vi "Vacuum Manual Control.vi"() -> ()   [LabVIEW 2017]
uses:
  Shared Components/Gantry Class/Gantry Class.lvclass
  Shared Components/WorkTable Class/WorkTable Class.lvclass
panel:
  out "error out":errorcluster
  in  "Module Chuck 5-slot 4 status":bool=TRUE
  in  "Module Chuck 5-slot 3 status":bool=TRUE
  in  "Module Chuck 5-slot 2 status":bool=TRUE
  in  "Module Chuck 5-slot 1 status":bool=TRUE
  in  "Module Chuck 4-slot 4 status":bool=TRUE
  in  "Module Chuck 4-slot 3 status":bool=TRUE
  in  "Module Chuck 4-slot 2 status":bool=TRUE
  in  "Module Chuck 4-slot 1 status":bool=TRUE
  in  "Module Chuck 3 status":bool=TRUE
  in  "Module Chuck 2 status":bool=TRUE
  in  "Module Chuck 1 status":bool=TRUE
  in  "Weight Chuck status":bool=TRUE
  in  "Stamp Chuck status":bool=TRUE
  in  "Glue Resevoir Chuck status":bool=TRUE
  in  "Outer Gantry Head status":bool=TRUE
  in  "Inner Gantry Head status":bool=TRUE
  in  "Reset all to ON":bool
  in  "Reset all to OFF":bool
  in  "stop program":bool
  in  "Virtual Mode":bool
  in  "Config Folder":path=path "C:/Users/husker/Desktop/gantry/Config"
  # "Note:\nMay not always read the correct initial vacuum states, due to incorrect reading of the worktable.\nIf in doubt, change all to off!"
  # "Current\nState"
  # "Vacuum\nChannel"
  # "Inner Gantry Head"
  # "Outer Gantry Head"
  # "Glue Resevoir Chuck"
  # "Stamp Chuck"
  # "Weight Chuck"
  # "Module Chuck 1"
  # "Module Chuck 2"
  # "Module Chuck 3"
  # "Module Chuck 4\n\nSlot 1\n\nSlot 2\n\nSlot 3\n\nSlot 4"
  # "Module Chuck 5\n\nSlot 1\n\nSlot 2\n\nSlot 3\n\nSlot 4"
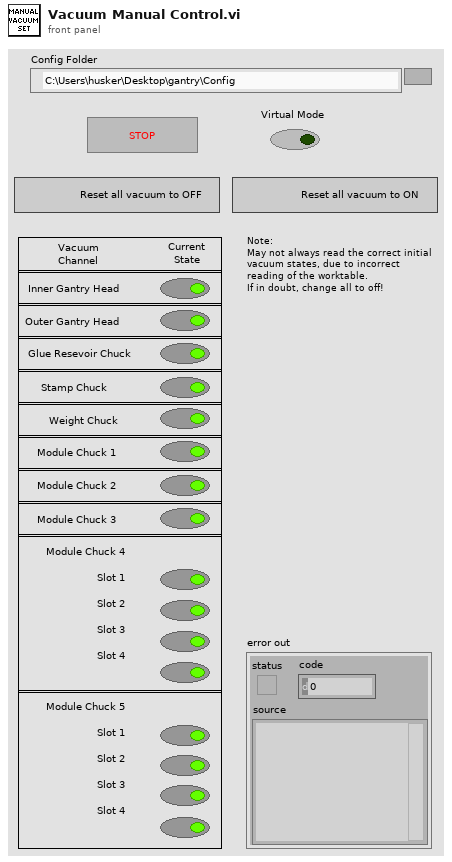
[diagram p1: front panel]
types:
  T1 = typedef "Worktable_Manifold.ctl" = cluster{"Vacuum Channel Status":T2[], "Vacuum Channel Names":T3[]}
  T2 = typedef "Worktable_Manifold Channel.ctl" = cluster{"Enabled":bool, "Hardware Path":string}
  T3 = typedef "Worktable_Manifold Channel Names.ctl" = cluster{"Channel Name":string, "Channel Number":i8}
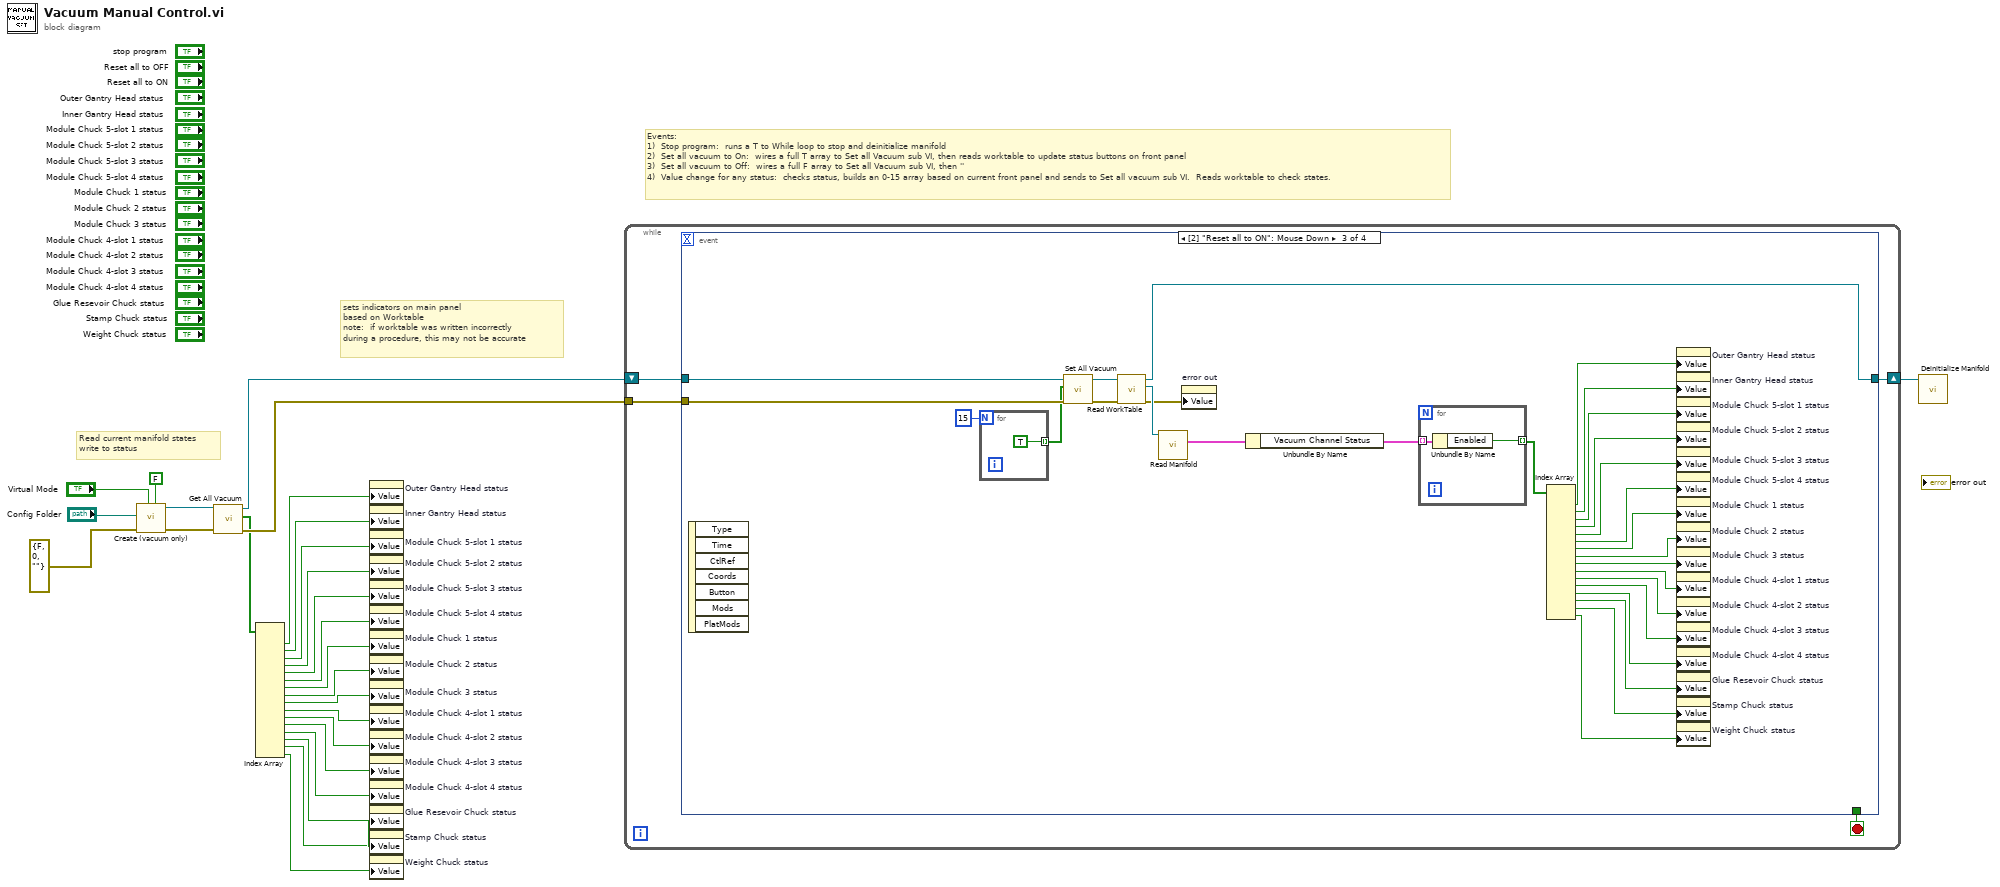
[diagram p0: block diagram]
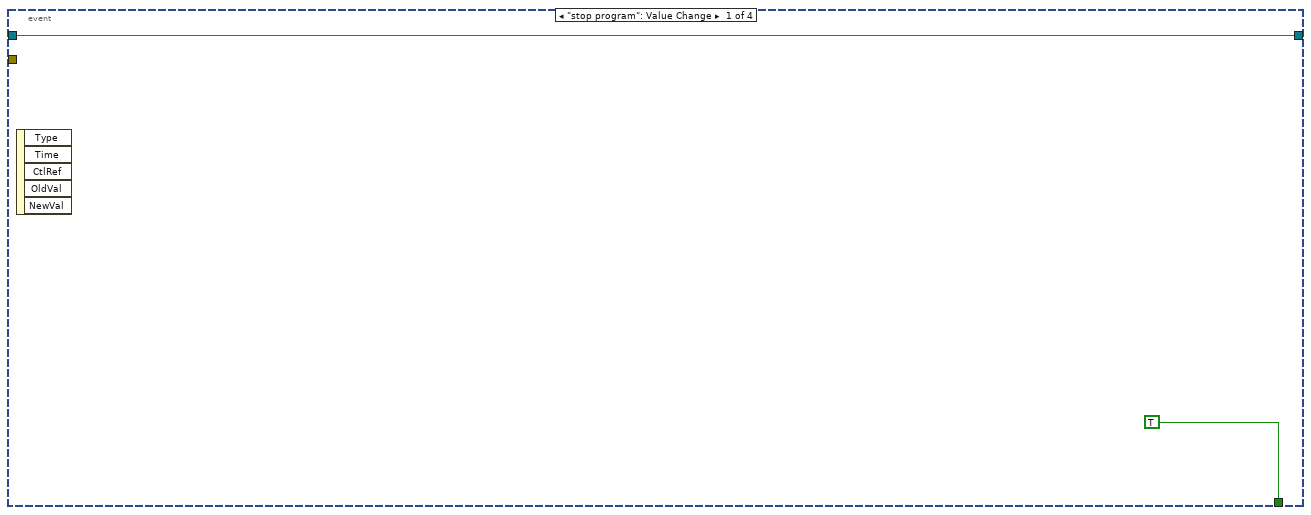
[diagram p2: hidden frame]
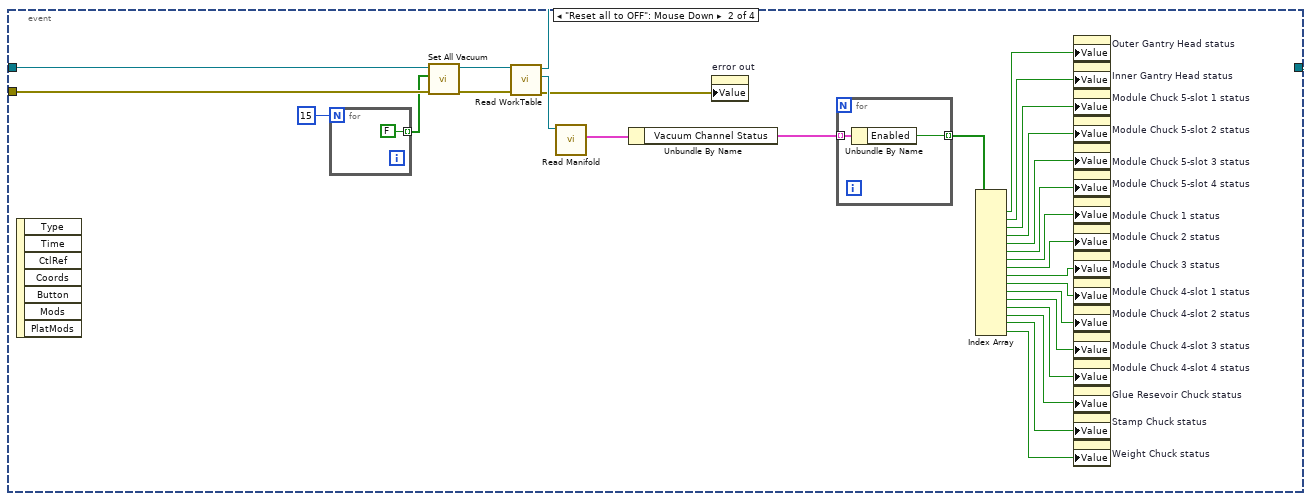
[diagram p3: hidden frame]
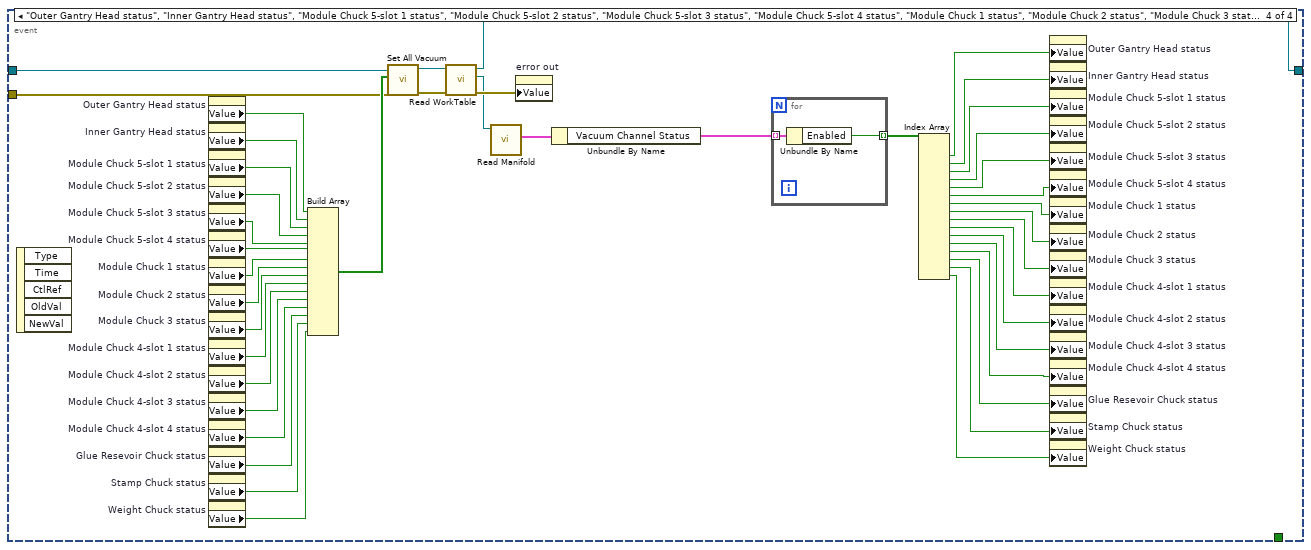
[diagram p4: hidden frame]
diagram:
  # "Events:\n1)  Stop program:  runs a T to While loop to stop and deinitialize manifold\n2)  Set all vacuum to On:  wires a full T array to Set all Vacuum sub VI, then reads worktable to update status buttons on front panel\n3)  Set all vacuum to Off:  wires a full F array to Set all Vacuum sub VI, then ''\n4)  Value change for any status:  checks status, builds an 0-15 array based on current front panel and sends to Set all vacuum sub VI.  Reads worktable to check states."
  # "sets indicators on main panel\nbased on Worktable\nnote:  if worktable was written incorrectly\nduring a procedure, this may not be accurate"
  # "Read current manifold states\nwrite to status"
  n1 = call "Create (vacuum only).vi"("Reset Vacuum to All Off?"=FALSE, "Virtual Mode"="Virtual Mode", "error in"=errorcluster {"status"=FALSE, "code"=0, "source"=""}, "Config Folder"="Config Folder") -> ("error out"=w14:errorcluster, "Gantry out"=w15:refnum<class "Gantry Class.lvclass">)  [unwired: 6 in]
  n2 = call "Get All Vacuum.vi"("error in"=w14, "Gantry Class in"=w15) -> ("error out"=w12:errorcluster, "Channel Array"=w11:bool[], "Gantry Class out"=w13:refnum<class "Gantry Class.lvclass">)  [unwired: 7 in]
  n3 = Index Array(array=w11) -> (element #1=w22:bool, element #2=w21:bool, element #3=w20:bool, element #4=w19:bool, element #5=w18:bool, element #6=w17:bool, element #7=w10:bool, element #8=w9:bool, element #9=w8:bool, element #10=w7:bool, element #11=w6:bool, element #12=w5:bool, element #13=w4:bool, element #14=w3:bool, element #15=w2:bool, element #16=w1:bool)  [unwired: 16 in]
  n4 = property on="Outer Gantry Head status" class="Bool (strict)"("Value"=w22) -> ()  [unwired: 2 in, 2 out]
  n5 = property on="Inner Gantry Head status" class="Bool (strict)"("Value"=w21) -> ()  [unwired: 2 in, 2 out]
  n6 = property on="Module Chuck 5-slot 1 status" class="Bool (strict)"("Value"=w20) -> ()  [unwired: 2 in, 2 out]
  n7 = property on="Module Chuck 5-slot 2 status" class="Bool (strict)"("Value"=w19) -> ()  [unwired: 2 in, 2 out]
  n8 = property on="Module Chuck 5-slot 3 status" class="Bool (strict)"("Value"=w18) -> ()  [unwired: 2 in, 2 out]
  n9 = property on="Module Chuck 5-slot 4 status" class="Bool (strict)"("Value"=w17) -> ()  [unwired: 2 in, 2 out]
  n10 = property on="Module Chuck 1 status" class="Bool (strict)"("Value"=w10) -> ()  [unwired: 2 in, 2 out]
  n11 = property on="Module Chuck 2 status" class="Bool (strict)"("Value"=w9) -> ()  [unwired: 2 in, 2 out]
  n12 = property on="Module Chuck 3 status" class="Bool (strict)"("Value"=w8) -> ()  [unwired: 2 in, 2 out]
  n13 = property on="Module Chuck 4-slot 1 status" class="Bool (strict)"("Value"=w7) -> ()  [unwired: 2 in, 2 out]
  n14 = property on="Module Chuck 4-slot 2 status" class="Bool (strict)"("Value"=w6) -> ()  [unwired: 2 in, 2 out]
  n15 = property on="Module Chuck 4-slot 3 status" class="Bool (strict)"("Value"=w5) -> ()  [unwired: 2 in, 2 out]
  n16 = property on="Module Chuck 4-slot 4 status" class="Bool (strict)"("Value"=w4) -> ()  [unwired: 2 in, 2 out]
  n17 = property on="Glue Resevoir Chuck status" class="Bool (strict)"("Value"=w3) -> ()  [unwired: 2 in, 2 out]
  n18 = property on="Stamp Chuck status" class="Bool (strict)"("Value"=w2) -> ()  [unwired: 2 in, 2 out]
  n19 = property on="Weight Chuck status" class="Bool (strict)"("Value"=w1) -> ()  [unwired: 2 in, 2 out]
  n20 = while {
    tunnel: w12 -> [w28]
    shift-right: [w27] -> w16
    shift-left: w13 -> [w29]
    stop <- w30 stop-if-true
    n21 = event shown="[2] \"Reset all to ON\": Mouse Down" {
      selector: _ -> [_ _ _ _]
      dyn-events: _ -> [_ _ _ _]
      timeout: _ -> [_ _ _ _]
      tunnel: [TRUE _ _ _] -> w30
      tunnel: w29 -> [w31 w49 w80 w126]
      tunnel: w28 -> [_ w48 w79 w106]
      tunnel: [w31 w50 w78 w124] -> w27
      event "stop program": Value Change {
        n22 = event-data() -> ()  [unwired: 1 in, 5 out]
      }
      event "Reset all to OFF": Mouse Down {
        n23 = event-data() -> ()  [unwired: 1 in, 7 out]
        n24 = for {
          N: 15 -> [_]
          tunnel: [FALSE ("On/Off")] -> w46 mode=indexing
        }
        n25 = call "Set All Vacuum.vi"("error in"=w48, "Channel Array"=w46, "Gantry Class in"=w49) -> ("error out"=w44:errorcluster, "Gantry Class out"=w45:refnum<class "Gantry Class.lvclass">)  [unwired: 7 in]
        n26 = call-dynamic "Read WorkTable.vi"("error in"=w44, "Gantry Class in"=w45) -> ("error out"=w51:errorcluster, "WorkTable Class.lvclass"=w58:refnum<class "WorkTable Class.lvclass">, "Gantry Class out"=w50:refnum<class "Gantry Class.lvclass">)  [unwired: 7 in]
        n27 = call-dynamic "Read Manifold.vi"("WorkTable Class in"=w58) -> ("Manifold"=w60:T1)  [unwired: 8 in, 2 out]
        n28 = Unbundle By Name(w60) -> ("Vacuum Channel Status"=w59:T2[])
        n29 = property on="error out" class="Clust (strict)"("Value"=w51) -> ()  [unwired: 2 in, 2 out]
        n30 = for {
          tunnel: w59 -> [w63] mode=indexing
          tunnel: [w62] -> w43 mode=indexing
          n31 = Unbundle By Name(w63) -> ("Enabled"=w62:bool)
        }
        n32 = Index Array(array=w43) -> (element #1=w57:bool, element #2=w56:bool, element #3=w55:bool, element #4=w54:bool, element #5=w53:bool, element #6=w52:bool, element #7=w42:bool, element #8=w41:bool, element #9=w40:bool, element #10=w39:bool, element #11=w38:bool, element #12=w37:bool, element #13=w36:bool, element #14=w35:bool, element #15=w34:bool, element #16=w33:bool)  [unwired: 16 in]
        n33 = property on="Outer Gantry Head status" class="Bool (strict)"("Value"=w57) -> ()  [unwired: 2 in, 2 out]
        n34 = property on="Inner Gantry Head status" class="Bool (strict)"("Value"=w56) -> ()  [unwired: 2 in, 2 out]
        n35 = property on="Module Chuck 5-slot 1 status" class="Bool (strict)"("Value"=w55) -> ()  [unwired: 2 in, 2 out]
        n36 = property on="Module Chuck 5-slot 2 status" class="Bool (strict)"("Value"=w54) -> ()  [unwired: 2 in, 2 out]
        n37 = property on="Module Chuck 5-slot 3 status" class="Bool (strict)"("Value"=w53) -> ()  [unwired: 2 in, 2 out]
        n38 = property on="Module Chuck 5-slot 4 status" class="Bool (strict)"("Value"=w52) -> ()  [unwired: 2 in, 2 out]
        n39 = property on="Module Chuck 1 status" class="Bool (strict)"("Value"=w42) -> ()  [unwired: 2 in, 2 out]
        n40 = property on="Module Chuck 2 status" class="Bool (strict)"("Value"=w41) -> ()  [unwired: 2 in, 2 out]
        n41 = property on="Module Chuck 3 status" class="Bool (strict)"("Value"=w40) -> ()  [unwired: 2 in, 2 out]
        n42 = property on="Module Chuck 4-slot 1 status" class="Bool (strict)"("Value"=w39) -> ()  [unwired: 2 in, 2 out]
        n43 = property on="Module Chuck 4-slot 2 status" class="Bool (strict)"("Value"=w38) -> ()  [unwired: 2 in, 2 out]
        n44 = property on="Module Chuck 4-slot 3 status" class="Bool (strict)"("Value"=w37) -> ()  [unwired: 2 in, 2 out]
        n45 = property on="Module Chuck 4-slot 4 status" class="Bool (strict)"("Value"=w36) -> ()  [unwired: 2 in, 2 out]
        n46 = property on="Glue Resevoir Chuck status" class="Bool (strict)"("Value"=w35) -> ()  [unwired: 2 in, 2 out]
        n47 = property on="Stamp Chuck status" class="Bool (strict)"("Value"=w34) -> ()  [unwired: 2 in, 2 out]
        n48 = property on="Weight Chuck status" class="Bool (strict)"("Value"=w33) -> ()  [unwired: 2 in, 2 out]
      }
      event "Reset all to ON": Mouse Down {
        n49 = event-data() -> ()  [unwired: 1 in, 7 out]
        n50 = for {
          N: 15 -> [_]
          tunnel: [TRUE ("On/Off")] -> w76 mode=indexing
        }
        n51 = call "Set All Vacuum.vi"("error in"=w79, "Channel Array"=w76, "Gantry Class in"=w80) -> ("error out"=w81:errorcluster, "Gantry Class out"=w82:refnum<class "Gantry Class.lvclass">)  [unwired: 7 in]
        n52 = call-dynamic "Read WorkTable.vi"("error in"=w81, "Gantry Class in"=w82) -> ("error out"=w75:errorcluster, "WorkTable Class.lvclass"=w89:refnum<class "WorkTable Class.lvclass">, "Gantry Class out"=w78:refnum<class "Gantry Class.lvclass">)  [unwired: 7 in]
        n53 = call-dynamic "Read Manifold.vi"("WorkTable Class in"=w89) -> ("Manifold"=w91:T1)  [unwired: 8 in, 2 out]
        n54 = property on="error out" class="Clust (strict)"("Value"=w75) -> ()  [unwired: 2 in, 2 out]
        n55 = Unbundle By Name(w91) -> ("Vacuum Channel Status"=w90:T2[])
        n56 = for {
          tunnel: w90 -> [w94] mode=indexing
          tunnel: [w93] -> w74 mode=indexing
          n57 = Unbundle By Name(w94) -> ("Enabled"=w93:bool)
        }
        n58 = Index Array(array=w74) -> (element #1=w88:bool, element #2=w87:bool, element #3=w86:bool, element #4=w85:bool, element #5=w84:bool, element #6=w83:bool, element #7=w73:bool, element #8=w72:bool, element #9=w71:bool, element #10=w70:bool, element #11=w69:bool, element #12=w68:bool, element #13=w67:bool, element #14=w66:bool, element #15=w65:bool, element #16=w64:bool)  [unwired: 16 in]
        n59 = property on="Outer Gantry Head status" class="Bool (strict)"("Value"=w88) -> ()  [unwired: 2 in, 2 out]
        n60 = property on="Inner Gantry Head status" class="Bool (strict)"("Value"=w87) -> ()  [unwired: 2 in, 2 out]
        n61 = property on="Module Chuck 5-slot 1 status" class="Bool (strict)"("Value"=w86) -> ()  [unwired: 2 in, 2 out]
        n62 = property on="Module Chuck 5-slot 2 status" class="Bool (strict)"("Value"=w85) -> ()  [unwired: 2 in, 2 out]
        n63 = property on="Module Chuck 5-slot 3 status" class="Bool (strict)"("Value"=w84) -> ()  [unwired: 2 in, 2 out]
        n64 = property on="Module Chuck 5-slot 4 status" class="Bool (strict)"("Value"=w83) -> ()  [unwired: 2 in, 2 out]
        n65 = property on="Module Chuck 1 status" class="Bool (strict)"("Value"=w73) -> ()  [unwired: 2 in, 2 out]
        n66 = property on="Module Chuck 2 status" class="Bool (strict)"("Value"=w72) -> ()  [unwired: 2 in, 2 out]
        n67 = property on="Module Chuck 3 status" class="Bool (strict)"("Value"=w71) -> ()  [unwired: 2 in, 2 out]
        n68 = property on="Module Chuck 4-slot 1 status" class="Bool (strict)"("Value"=w70) -> ()  [unwired: 2 in, 2 out]
        n69 = property on="Module Chuck 4-slot 2 status" class="Bool (strict)"("Value"=w69) -> ()  [unwired: 2 in, 2 out]
        n70 = property on="Module Chuck 4-slot 3 status" class="Bool (strict)"("Value"=w68) -> ()  [unwired: 2 in, 2 out]
        n71 = property on="Module Chuck 4-slot 4 status" class="Bool (strict)"("Value"=w67) -> ()  [unwired: 2 in, 2 out]
        n72 = property on="Glue Resevoir Chuck status" class="Bool (strict)"("Value"=w66) -> ()  [unwired: 2 in, 2 out]
        n73 = property on="Stamp Chuck status" class="Bool (strict)"("Value"=w65) -> ()  [unwired: 2 in, 2 out]
        n74 = property on="Weight Chuck status" class="Bool (strict)"("Value"=w64) -> ()  [unwired: 2 in, 2 out]
      }
      event "Outer Gantry Head status", "Inner Gantry Head status", "Module Chuck 5-slot 1 status", "Module Chuck 5-slot 2 status", "Module Chuck 5-slot 3 status", "Module Chuck 5-slot 4 status", "Module Chuck 1 status", "Module Chuck 2 status", "Module Chuck 3 status", "Module Chuck 4-slot 1 status", "Module Chuck 4-slot 2 status", "Module Chuck 4-slot 3 status", "Module Chuck 4-slot 4 status", "Glue Resevoir Chuck status", "Stamp Chuck status", "Weight Chuck status": Value Change {
        n75 = event-data() -> ()  [unwired: 1 in, 5 out]
        n76 = property on="Outer Gantry Head status" class="Bool (strict)"() -> ("Value"=w123:bool)  [unwired: 2 in, 2 out]
        n77 = property on="Inner Gantry Head status" class="Bool (strict)"() -> ("Value"=w122:bool)  [unwired: 2 in, 2 out]
        n78 = property on="Module Chuck 5-slot 1 status" class="Bool (strict)"() -> ("Value"=w121:bool)  [unwired: 2 in, 2 out]
        n79 = property on="Module Chuck 5-slot 2 status" class="Bool (strict)"() -> ("Value"=w120:bool)  [unwired: 2 in, 2 out]
        n80 = property on="Module Chuck 5-slot 3 status" class="Bool (strict)"() -> ("Value"=w119:bool)  [unwired: 2 in, 2 out]
        n81 = property on="Module Chuck 5-slot 4 status" class="Bool (strict)"() -> ("Value"=w118:bool)  [unwired: 2 in, 2 out]
        n82 = property on="Module Chuck 1 status" class="Bool (strict)"() -> ("Value"=w117:bool)  [unwired: 2 in, 2 out]
        n83 = property on="Module Chuck 2 status" class="Bool (strict)"() -> ("Value"=w116:bool)  [unwired: 2 in, 2 out]
        n84 = property on="Module Chuck 3 status" class="Bool (strict)"() -> ("Value"=w115:bool)  [unwired: 2 in, 2 out]
        n85 = property on="Module Chuck 4-slot 1 status" class="Bool (strict)"() -> ("Value"=w114:bool)  [unwired: 2 in, 2 out]
        n86 = property on="Module Chuck 4-slot 2 status" class="Bool (strict)"() -> ("Value"=w113:bool)  [unwired: 2 in, 2 out]
        n87 = property on="Module Chuck 4-slot 3 status" class="Bool (strict)"() -> ("Value"=w112:bool)  [unwired: 2 in, 2 out]
        n88 = property on="Module Chuck 4-slot 4 status" class="Bool (strict)"() -> ("Value"=w111:bool)  [unwired: 2 in, 2 out]
        n89 = property on="Glue Resevoir Chuck status" class="Bool (strict)"() -> ("Value"=w110:bool)  [unwired: 2 in, 2 out]
        n90 = property on="Stamp Chuck status" class="Bool (strict)"() -> ("Value"=w109:bool)  [unwired: 2 in, 2 out]
        n91 = property on="Weight Chuck status" class="Bool (strict)"() -> ("Value"=w108:bool)  [unwired: 2 in, 2 out]
        n92 = Build Array(w123, w122, w121, w120, w119, w118, w117, w116, w115, w114, w113, w112, w111, w110, w109, w108) -> (w107:bool[])
        n93 = call "Set All Vacuum.vi"("error in"=w106, "Channel Array"=w107, "Gantry Class in"=w126) -> ("error out"=w136:errorcluster, "Gantry Class out"=w135:refnum<class "Gantry Class.lvclass">)  [unwired: 7 in]
        n94 = call-dynamic "Read WorkTable.vi"("error in"=w136, "Gantry Class in"=w135) -> ("error out"=w137:errorcluster, "WorkTable Class.lvclass"=w129:refnum<class "WorkTable Class.lvclass">, "Gantry Class out"=w124:refnum<class "Gantry Class.lvclass">)  [unwired: 7 in]
        n95 = call-dynamic "Read Manifold.vi"("WorkTable Class in"=w129) -> ("Manifold"=w127:T1)  [unwired: 8 in, 2 out]
        n96 = property on="error out" class="Clust (strict)"("Value"=w137) -> ()  [unwired: 2 in, 2 out]
        n97 = Unbundle By Name(w127) -> ("Vacuum Channel Status"=w128:T2[])
        n98 = for {
          tunnel: w128 -> [w139] mode=indexing
          tunnel: [w138] -> w125 mode=indexing
          n99 = Unbundle By Name(w139) -> ("Enabled"=w138:bool)
        }
        n100 = Index Array(array=w125) -> (element #1=w130:bool, element #2=w131:bool, element #3=w132:bool, element #4=w133:bool, element #5=w134:bool, element #6=w105:bool, element #7=w104:bool, element #8=w103:bool, element #9=w102:bool, element #10=w101:bool, element #11=w100:bool, element #12=w99:bool, element #13=w98:bool, element #14=w97:bool, element #15=w96:bool, element #16=w95:bool)  [unwired: 16 in]
        n101 = property on="Outer Gantry Head status" class="Bool (strict)"("Value"=w130) -> ()  [unwired: 2 in, 2 out]
        n102 = property on="Inner Gantry Head status" class="Bool (strict)"("Value"=w131) -> ()  [unwired: 2 in, 2 out]
        n103 = property on="Module Chuck 5-slot 1 status" class="Bool (strict)"("Value"=w132) -> ()  [unwired: 2 in, 2 out]
        n104 = property on="Module Chuck 5-slot 2 status" class="Bool (strict)"("Value"=w133) -> ()  [unwired: 2 in, 2 out]
        n105 = property on="Module Chuck 5-slot 3 status" class="Bool (strict)"("Value"=w134) -> ()  [unwired: 2 in, 2 out]
        n106 = property on="Module Chuck 5-slot 4 status" class="Bool (strict)"("Value"=w105) -> ()  [unwired: 2 in, 2 out]
        n107 = property on="Module Chuck 1 status" class="Bool (strict)"("Value"=w104) -> ()  [unwired: 2 in, 2 out]
        n108 = property on="Module Chuck 2 status" class="Bool (strict)"("Value"=w103) -> ()  [unwired: 2 in, 2 out]
        n109 = property on="Module Chuck 3 status" class="Bool (strict)"("Value"=w102) -> ()  [unwired: 2 in, 2 out]
        n110 = property on="Module Chuck 4-slot 1 status" class="Bool (strict)"("Value"=w101) -> ()  [unwired: 2 in, 2 out]
        n111 = property on="Module Chuck 4-slot 2 status" class="Bool (strict)"("Value"=w100) -> ()  [unwired: 2 in, 2 out]
        n112 = property on="Module Chuck 4-slot 3 status" class="Bool (strict)"("Value"=w99) -> ()  [unwired: 2 in, 2 out]
        n113 = property on="Module Chuck 4-slot 4 status" class="Bool (strict)"("Value"=w98) -> ()  [unwired: 2 in, 2 out]
        n114 = property on="Glue Resevoir Chuck status" class="Bool (strict)"("Value"=w97) -> ()  [unwired: 2 in, 2 out]
        n115 = property on="Stamp Chuck status" class="Bool (strict)"("Value"=w96) -> ()  [unwired: 2 in, 2 out]
        n116 = property on="Weight Chuck status" class="Bool (strict)"("Value"=w95) -> ()  [unwired: 2 in, 2 out]
      }
    }
  }
  n117 = call-dynamic "Deinitialize Manifold.vi"("Gantry Class in"=w16) -> ()  [unwired: 9 in, 2 out]
